vi "Create Virtual Folder.vi"(7 "Curent Bus Path":path, 8 "error in":errorcluster, 9 "Bus Number":i32, 10 "Virtual Folder Name":string, 11 "Path to Project":path) -> (0 "error out":errorcluster, 1 "FPGA Target Found":bool, 2 "New Virtual Folder":refnum<vi>, 3 "Project:Open":refnum<vi>)   [LabVIEW 2014, in "Initialization and IO Node Scripting.lvlib"]
uses:
  Initialization and IO Node Scripting.lvlib
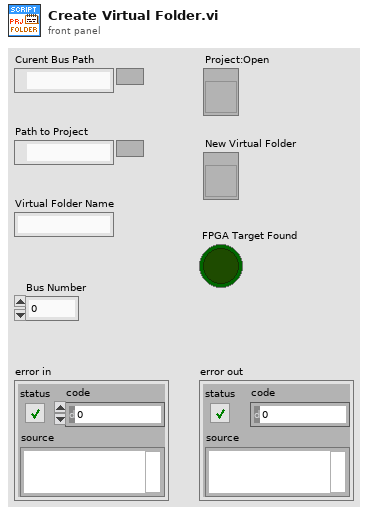
[diagram p1: front panel]
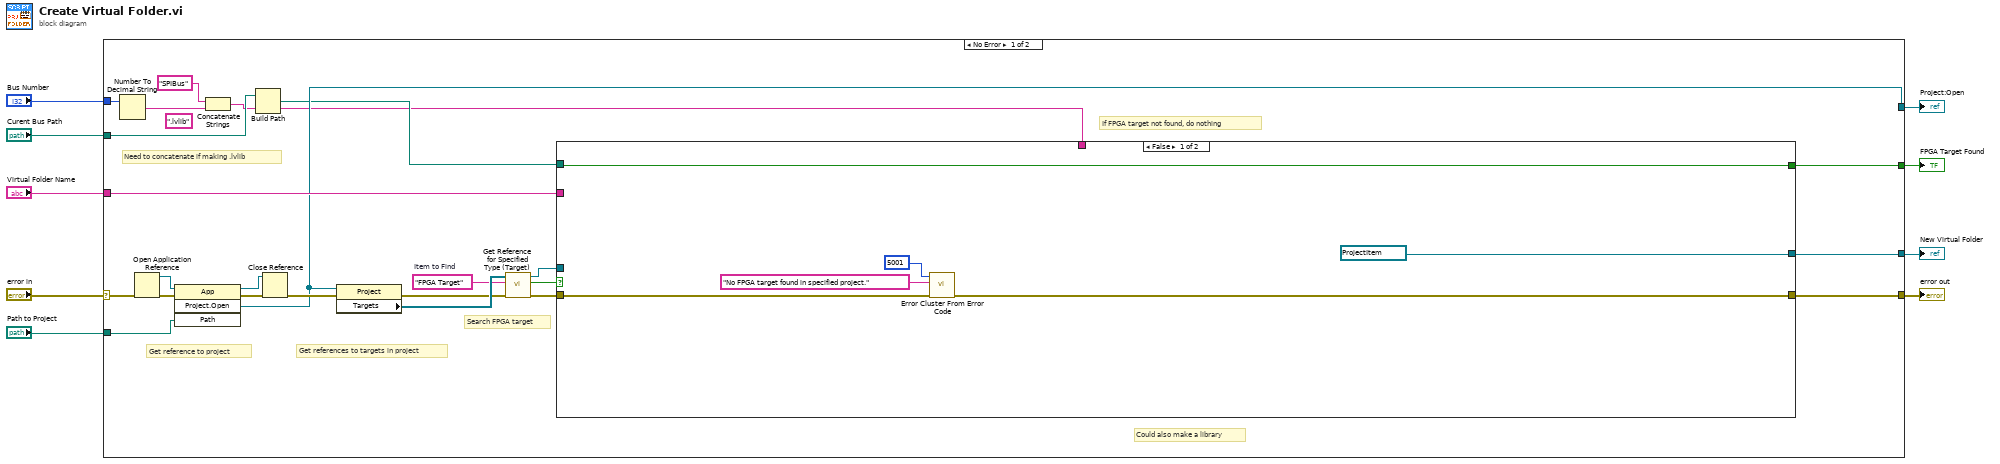
[diagram p0: block diagram]
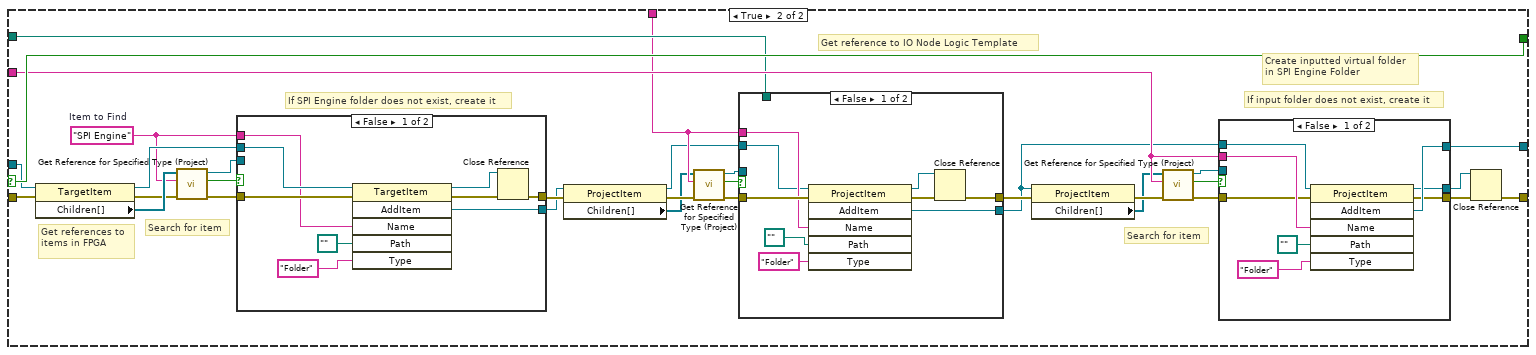
[diagram p2: hidden frame]
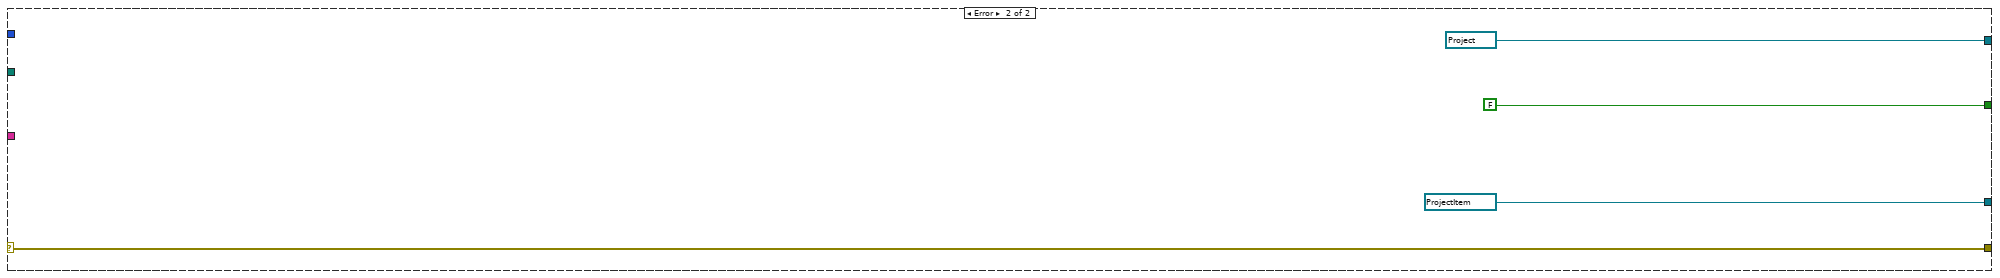
[diagram p6: hidden frame]
diagram:
  n1 = case shown="No Error" "error in" {
    selector: "error in" -> [w28 w105]
    tunnel: "Path to Project" -> [w31 _]
    tunnel: [w25 w105] -> w7
    tunnel: [w23 FALSE] -> w6
    tunnel: "Virtual Folder Name" -> [w22 _]
    tunnel: [w19 refnum<vi> refnum ("Project:Open")] -> w4
    tunnel: [w18 refnum<vi> refnum ("Project Item")] -> w3
    tunnel: "Bus Number" -> [w15 _]
    tunnel: "Curent Bus Path" -> [w14 _]
    frame No Error {
      (unwired) ".lvlib" ("string")
      w32 = "FPGA Target"  # Item to Find
      # "Need to concatenate if making .lvlib"
      # "Could also make a library"
      # "Search FPGA target"
      # "If FPGA target not found, do nothing"
      # "Get references to targets in project"
      # "Get reference to project"
      n2 = Number To Decimal String(number=w15) -> (decimal integer string=w16:string)  [unwired: 1 in]
      n3 = Open Application Reference(8:w28) -> (0:w29:errorcluster, 3:w30:refnum<vi>)  [unwired: 3 in]
      n4 = invoke class="App" method="Project.Open"(reference=w30, error in=w29, "Path"=w31) -> (reference out=w10:refnum<vi>, error out=w13:errorcluster, "Project:Open"=w19:refnum<vi>)  [unwired: 1 in, 1 out]
      n5 = Concatenate Strings("SPIBus", w16) -> (w11:string)
      n6 = Build Path(base path=w14, name or relative path=w11) -> (appended path=w12:path)
      n7 = Close Reference(reference=w10, error in (no error)=w13) -> (error out=w20:errorcluster)
      n8 = property class="Project"(reference=w19, error in=w20) -> (error out=w21:errorcluster, "Targets"=w33:refnum<vi>[])  [unwired: 1 out]
      n9 = call "Get Reference for Specified Type (Target).vi"("error in (no error)"=w21, "Item to Find"=w32, "Array of References"=w33) -> ("error out"=w27:errorcluster, "Item Found"=w24:bool, "TargetItem out"=w26:refnum<vi>)  [unwired: 6 in]
      n10 = case shown="False" w24 {
        selector: w24 -> [w38 w67]
        tunnel: [refnum<vi> refnum ("AddItem") w71] -> w18
        tunnel: w27 -> [w34 w49]
        tunnel: w26 -> [_ w50]
        tunnel: [w35 w70] -> w25
        tunnel: [w38 w67] -> w23
        tunnel: w22 -> [_ w64]
        tunnel: w12 -> [_ w47]
        tunnel: w11 -> [_ w46]
        frame False {
          n11 = call <vilib>:"Error Cluster From Error Code.vi"("error in (no error)"=w34, "error message (\"\")"="No FPGA target found in specified project." ("error message (\"\")"), "error code (0)"=5001) -> ("error out"=w35:errorcluster)  [unwired: 6 in]
        }
        frame True {
          w52 = "SPI Engine"  # Item to Find
          # "Get reference to IO Node Logic Template"
          # "Search for item"
          # "Get references to items in FPGA"
          # "If SPI Engine folder does not exist, create it"
          # "Search for item"
          # "Create inputted virtual folder\nin SPI Engine Folder"
          # "If input folder does not exist, create it"
          n12 = property class="TargetItem"(reference=w50, error in=w49) -> (reference out=w53:refnum<vi>, error out=w54:errorcluster, "Children[]"=w58:refnum<vi>[])
          n13 = call "Get Reference for Specified Type (Project).vi"("error in (no error)"=w54, "Type to Find"=w52, "Array of References"=w58) -> ("error out"=w56:errorcluster, "Item Found"=w57:bool, "Project Item"=w55:refnum<vi>)  [unwired: 6 in]
          n14 = case shown="False" w57 {
            tunnel: [w89 w92] -> w48
            tunnel: w56 -> [w86 w93]
            tunnel: w55 -> [_ w92]
            tunnel: [w84 w93] -> w51
            tunnel: w53 -> [w85 _]
            tunnel: w52 -> [w83 _]
            frame False {
              n15 = invoke class="TargetItem" method="AddItem"(reference=w85, error in=w86, "Name"=w83, "Path"=path "", "Type"="Folder") -> (reference out=w91:refnum<vi>, error out=w90:errorcluster, "AddItem"=w89:refnum<vi>)  [unwired: 1 in, 3 out]
              n16 = Close Reference(reference=w91, error in (no error)=w90) -> (error out=w84:errorcluster)
            }
            frame True {
            }
          }
          n17 = property class="ProjectItem"(reference=w48, error in=w51) -> (reference out=w40:refnum<vi>, error out=w45:errorcluster, "Children[]"=w44:refnum<vi>[])
          n18 = call "Get Reference for Specified Type (Project).vi"("error in (no error)"=w45, "Type to Find"=w46, "Array of References"=w44) -> ("error out"=w42:errorcluster, "Item Found"=w43:bool, "Project Item"=w41:refnum<vi>)  [unwired: 6 in]
          n19 = case shown="False" w43 {
            tunnel: [w75 w81] -> w60
            tunnel: w42 -> [w80 w81]
            tunnel: w41 -> [_ w82]
            tunnel: [w74 w82] -> w59
            tunnel: w46 -> [w78 _]
            tunnel: w40 -> [w73 _]
            tunnel: w47 -> [_ _]
            frame False {
              n20 = invoke class="ProjectItem" method="AddItem"(reference=w73, error in=w80, "Name"=w78, "Path"=path "", "Type"="Folder") -> (reference out=w76:refnum<vi>, error out=w77:errorcluster, "AddItem"=w74:refnum<vi>)  [unwired: 1 in, 3 out]
              n21 = Close Reference(reference=w76, error in (no error)=w77) -> (error out=w75:errorcluster)
            }
            frame True {
            }
          }
          n22 = property class="ProjectItem"(reference=w59, error in=w60) -> (error out=w62:errorcluster, "Children[]"=w61:refnum<vi>[])  [unwired: 1 out]
          n23 = call "Get Reference for Specified Type (Project).vi"("error in (no error)"=w62, "Type to Find"=w64, "Array of References"=w61) -> ("error out"=w65:errorcluster, "Item Found"=w66:bool, "Project Item"=w63:refnum<vi>)  [unwired: 6 in]
          n24 = case shown="False" w66 {
            tunnel: [w101 w102] -> w71
            tunnel: w59 -> [w100 w104]
            tunnel: [w99 w104] -> w69
            tunnel: [w98 w103] -> w68
            tunnel: w65 -> [w94 w103]
            tunnel: w64 -> [w95 _]
            tunnel: w63 -> [_ w102]
            frame False {
              n25 = invoke class="ProjectItem" method="AddItem"(reference=w100, error in=w94, "Name"=w95, "Path"=path "", "Type"="Folder") -> (reference out=w99:refnum<vi>, error out=w98:errorcluster, "AddItem"=w101:refnum<vi>)  [unwired: 1 in, 3 out]
            }
            frame True {
            }
          }
          n26 = Close Reference(reference=w69, error in (no error)=w68) -> (error out=w70:errorcluster)
        }
      }
    }
    frame Error {
    }
  }
  "error out" <- w7
  "New Virtual Folder" <- w3
  "FPGA Target Found" <- w6
  "Project:Open" <- w4
